vi "数采仪日志报警存储(子VI).vi"   [LabVIEW 2016, in "数据传输系统.lvlib"]
types:
  T1 = cluster{"时间标识":timestamp, "设备":string, "日志信息":string, "流程参数":string}
  T2 = cluster{"时间标识":timestamp, "设备":string, "日志信息":string}
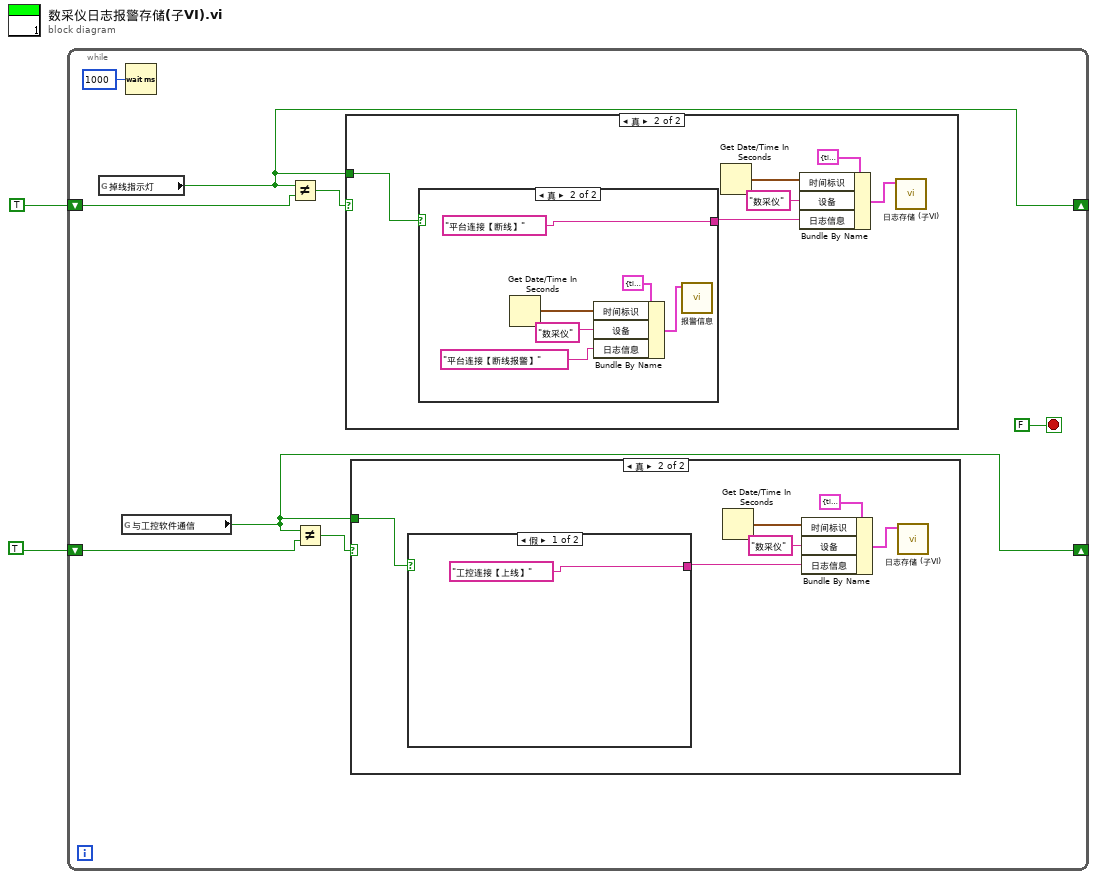
[diagram p0: block diagram]
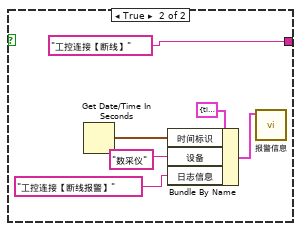
[diagram p3: hidden frame]
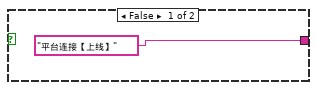
[diagram p5: hidden frame]
diagram:
  n1 = while {
    shift-right: [w6] -> _
    shift-left: TRUE -> [w7]
    shift-right: [w3] -> _
    shift-left: TRUE -> [w4]
    stop <- FALSE stop-if-true
    n2 = global read "全局 数据发送重叠.vi" "掉线指示灯"() -> (w6:bool)
    n3 = global read "全局1.vi" "与工控软件通信"() -> (w3:bool)
    n4 = Wait (ms)(milliseconds to wait=u32 1000 ("等待时间（毫秒）")) -> ()  [unwired: 1 out]
    n5 = Not Equal?(x=w6, y=w7) -> (x != y?=w8:bool)
    n6 = Not Equal?(x=w3, y=w4) -> (x != y?=w5:bool)
    n7 = case shown="真" w8 {
      tunnel: w6 -> [_ w24]
      frame False {
      }
      frame True {
        n8 = case shown="真" w24 {
          tunnel: ["平台连接【上线】" ("设备") "平台连接【断线】" ("设备")] -> w25
          frame False {
          }
          frame True {
            n9 = Get Date/Time In Seconds() -> (seconds since 1Jan1904=w33:timestamp)
            n10 = Bundle By Name(cluster=T2 {"时间标识"=timestamp(0 s since 1904-01-01), "设备"="", "日志信息"=""} ("data in"), "时间标识"=w33, "设备"="数采仪", "日志信息"="平台连接【断线报警】" ("设备")) -> (w34:T2)
            n11 = call "报警信息.vi"("data in"=w34) -> ()  [unwired: 10 in, 1 out]
          }
        }
        n12 = Get Date/Time In Seconds() -> (seconds since 1Jan1904=w27:timestamp)
        n13 = Bundle By Name(cluster=T1 {"时间标识"=timestamp(0 s since 1904-01-01), "设备"="", "日志信息"="", "流程参数"=""} ("data in"), "时间标识"=w27, "设备"="数采仪", "日志信息"=w25) -> (w28:T1)
        n14 = call "日志存储 (子VI).vi"("data in"=w28) -> ()  [unwired: 11 in]
      }
    }
    n15 = case shown="真" w5 {
      tunnel: w3 -> [_ w11]
      frame False {
      }
      frame True {
        n16 = case shown="假" w11 {
          tunnel: ["工控连接【上线】" ("设备") "工控连接【断线】" ("设备")] -> w12
          frame False {
          }
          frame True {
            n17 = Get Date/Time In Seconds() -> (seconds since 1Jan1904=w20:timestamp)
            n18 = Bundle By Name(cluster=T2 {"时间标识"=timestamp(0 s since 1904-01-01), "设备"="", "日志信息"=""} ("data in"), "时间标识"=w20, "设备"="数采仪", "日志信息"="工控连接【断线报警】" ("设备")) -> (w21:T2)
            n19 = call "报警信息.vi"("data in"=w21) -> ()  [unwired: 10 in, 1 out]
          }
        }
        n20 = Get Date/Time In Seconds() -> (seconds since 1Jan1904=w14:timestamp)
        n21 = Bundle By Name(cluster=T1 {"时间标识"=timestamp(0 s since 1904-01-01), "设备"="", "日志信息"="", "流程参数"=""} ("data in"), "时间标识"=w14, "设备"="数采仪", "日志信息"=w12) -> (w15:T1)
        n22 = call "日志存储 (子VI).vi"("data in"=w15) -> ()  [unwired: 11 in]
      }
    }
  }
